vi "getStatus.vi"(8 "error in (no error)":errorcluster, 11 "GenericMission in":refnum<class "GenericMission.lvclass">) -> (0 "error out":errorcluster, 2 "Status":string, 3 "GenericMission out":refnum<class "GenericMission.lvclass">)   [LabVIEW 2011, in "GenericMission.lvclass"]
uses:
  GenericMission.lvclass
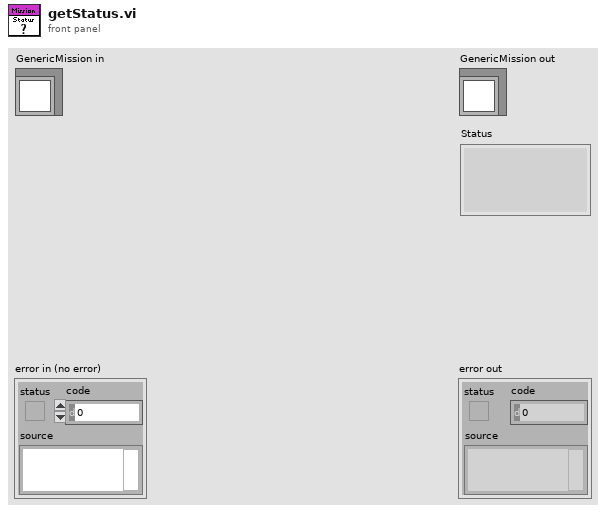
[diagram p1: front panel]
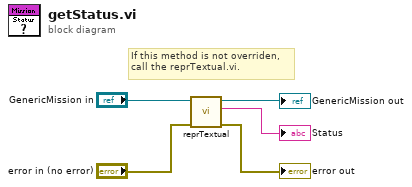
[diagram p0: block diagram]
diagram:
  # "If this method is not overriden,\ncall the reprTextual.vi."
  n1 = call-dynamic "reprTextual.vi"("error in (no error)"="error in (no error)", "GenericMission in"="GenericMission in") -> ("error out"=→"error out":errorcluster, "Description"=→"Status":string, "GenericMission out"=→"GenericMission out":refnum<class "GenericMission.lvclass">)  [unwired: 7 in]
